vi "Home.vi"(10 "error in (no error)":errorcluster) -> ()   [LabVIEW 2017]
uses:
  C:/X682 Camera Chassis Tester Program/data/Thorlabs.MotionControl.IntegratedStepperMotorsCLI.dll
  data/Thorlabs.MotionControl.IntegratedStepperMotorsCLI.dll
  C:/X682 Camera Chassis Tester Program/data/Thorlabs.MotionControl.Controls.dll
  data/Thorlabs.MotionControl.Controls.dll
panel:
  in  "SerialNumber":string
  in  "LongTravelStageControl":refnum<k24>(container)
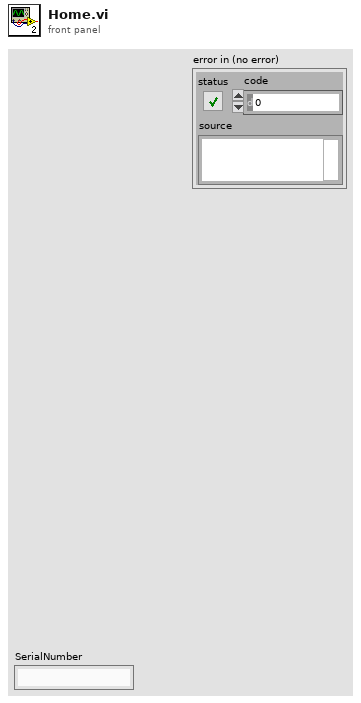
[diagram p1: front panel]
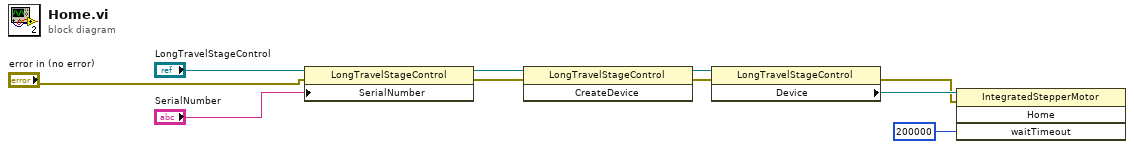
[diagram p0: block diagram]
diagram:
  n1 = property class="LongTravelStageControl"(reference="LongTravelStageControl", error in="error in (no error)", "SerialNumber"="SerialNumber") -> (reference out=w10:refnum<k24>, error out=w8:errorcluster)
  n2 = invoke class="LongTravelStageControl" method="CreateDevice"(reference=w10, error in=w8) -> (reference out=w9:refnum<k24>, error out=w7:errorcluster)  [unwired: 1 in, 1 out]
  n3 = property class="LongTravelStageControl"(reference=w9, error in=w7) -> (error out=w1:errorcluster, "Device"=w2:refnum<k24>)  [unwired: 1 out]
  n4 = invoke class="IntegratedStepperMotor" method="Home"(reference=w2, error in=w1, "waitTimeout"=200000) -> ()  [unwired: 1 in, 4 out]
